vi "tprofile_testread.vi"() -> ()   [LabVIEW 2017]
uses:
  <vilib>/Utility/file.llb/Read Delimited Spreadsheet (string).vi
panel:
  out "Array 4":i32[](array[numeric])
  out "Array 3":i32[](array[numeric])
  out "Array 2":i32[](array[numeric])
  out "output array":i32[](array[numeric])
  out "Array":i32[](array[numeric])
  out "all rows":string[][](array[string])
  in  "Path":path
  in  "stop":bool
  in  "Import Profile":bool
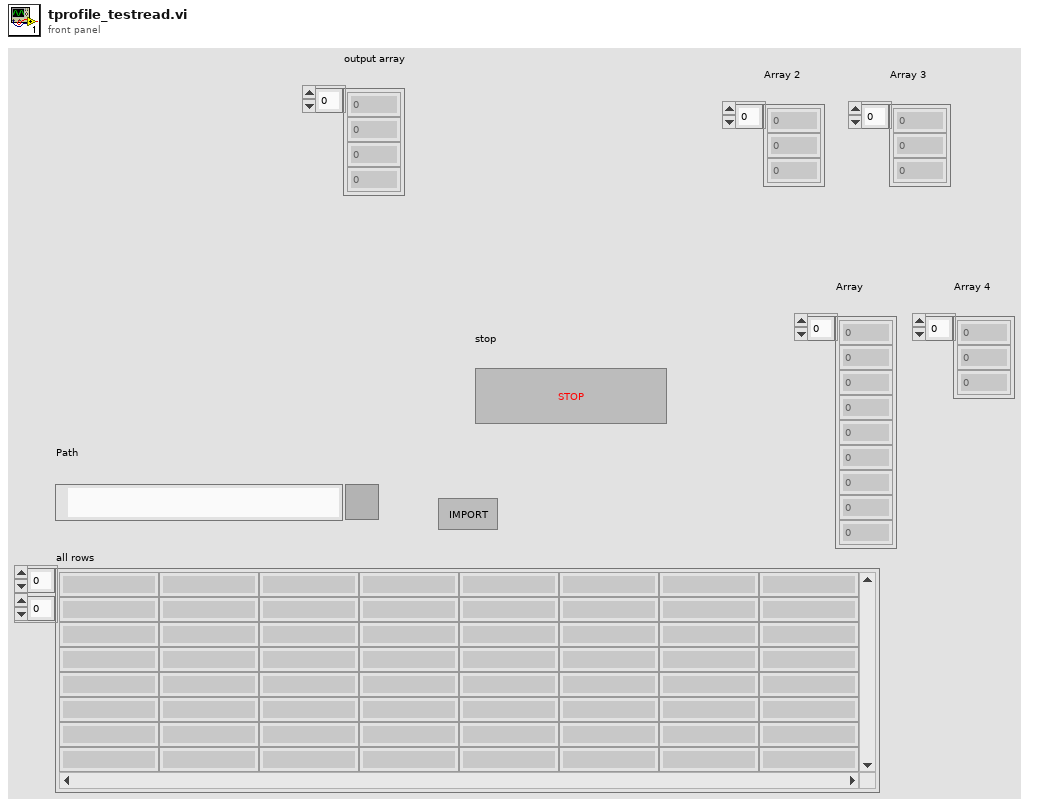
[diagram p1: front panel]
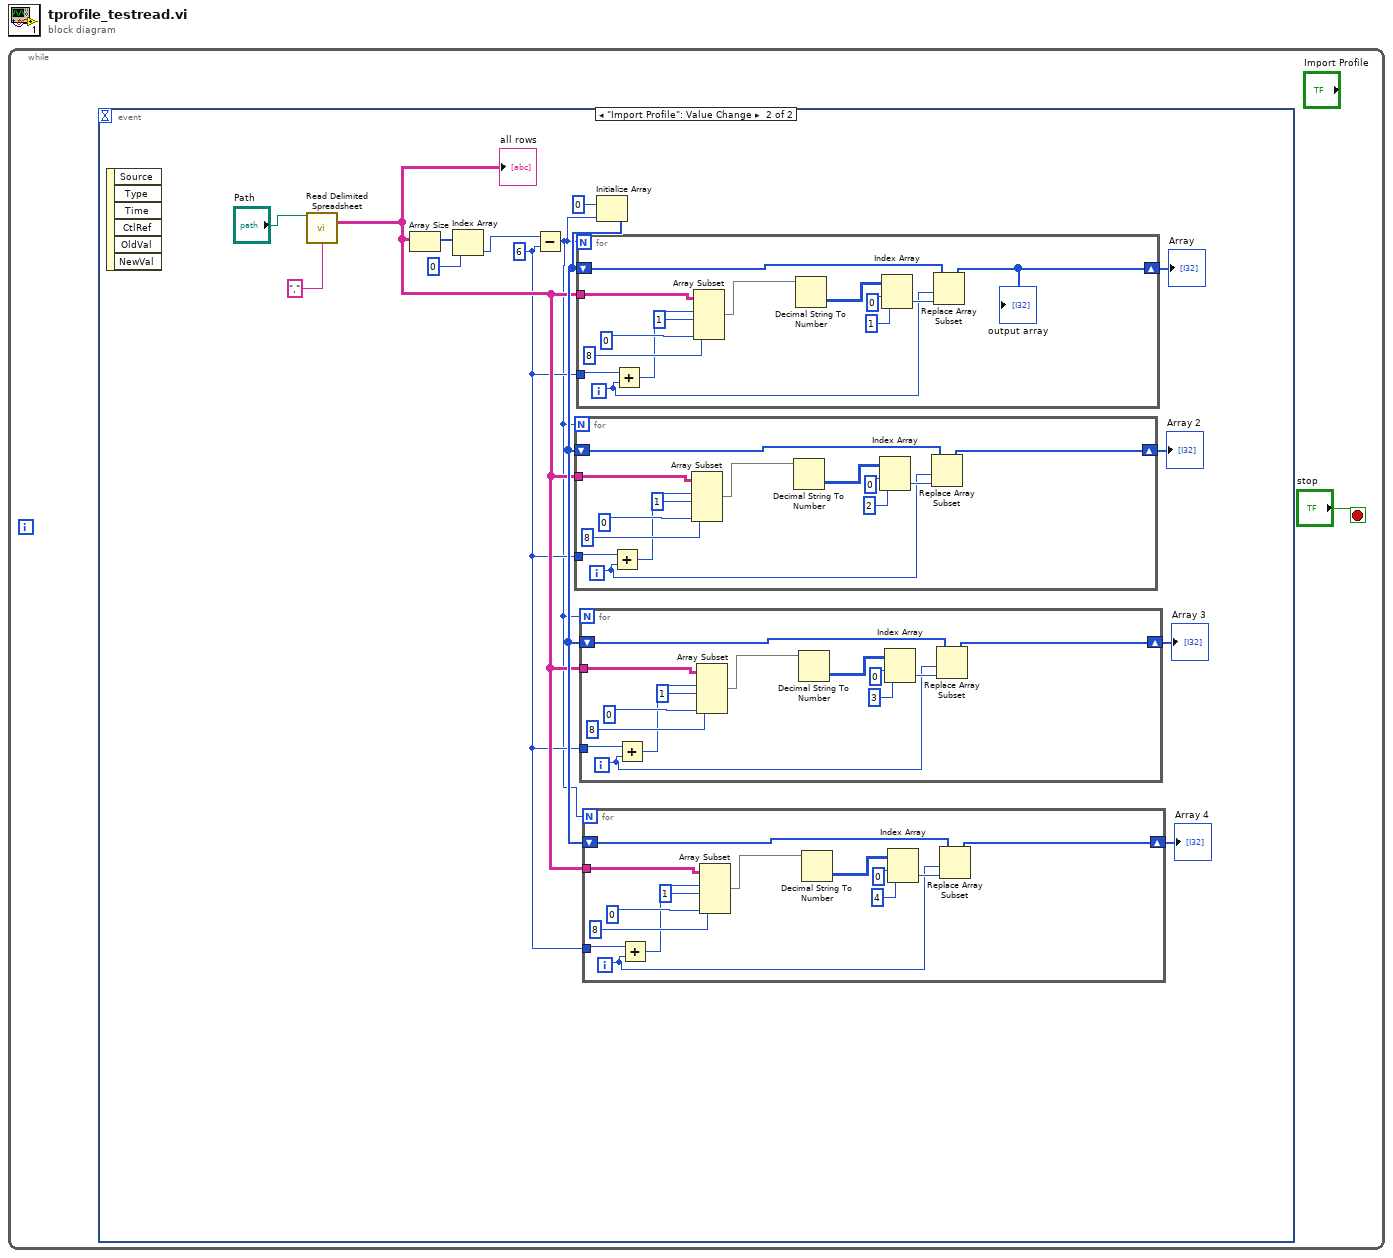
[diagram p0: block diagram]
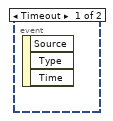
[diagram p2: hidden frame]
diagram:
  n1 = while {
    stop <- "stop" stop-if-true
    n2 = event shown="[1] \"Import Profile\": Value Change" {
      selector: _ -> [_ _]
      dyn-events: _ -> [_ _]
      timeout: _ -> [_ _]
      event Timeout {
        n3 = event-data() -> ()  [unwired: 1 in, 3 out]
      }
      event "Import Profile": Value Change {
        w3 = 6 ("Numeric")
        n4 = event-data() -> ()  [unwired: 1 in, 6 out]
        n5 = call-poly <vilib>:"Read Delimited Spreadsheet.vi"("file path (dialog if empty)"="Path", "delimiter (\\t)"="," ("delimiter (\\t)")) -> ("all rows"=w4:string[][])  [unwired: 8 in, 5 out]
        "all rows" <- w4
        n6 = Array Size(array=w4) -> (size(s)=w13:i32[])
        n7 = Index Array(array=w13, index=0) -> (element=w11:i32)
        n8 = Subtract(x=w11, y=w3) -> (x-y=w2:i32)
        n9 = Initialize Array(0, w2) -> (w5:i32[])
        n10 = for {
          N: w2 -> [_]
          tunnel: w4 -> [w57]
          tunnel: w3 -> [w52]
          shift-right: [w44] -> w8
          shift-left: w5 -> [w45]
          i -> [w47]
          n11 = Add(x=w52, y=w47) -> (x+y=w53:i32)
          n12 = Array Subset(array=w57, index (row)=w53, length (row)=1 ("length"), index (col)=0 ("index"), length (col)=8 ("length")) -> (w51:string[][])
          n13 = Decimal String To Number(string=w51) -> (number=w46:i32[][])  [unwired: 2 in, 1 out]
          n14 = Index Array(array=w46, index (row)=0, index (col)=2 ("disabled index (col)")) -> (element=w49:i32)
          n15 = Replace Array Subset(array=w45, new element=w49, index=w47) -> (w44:i32[])
        }
        "Array 2" <- w8
        n16 = for {
          N: w2 -> [_]
          tunnel: w4 -> [w71]
          tunnel: w3 -> [w66]
          shift-right: [w62] -> w9
          shift-left: w5 -> [w58]
          i -> [w60]
          n17 = Add(x=w66, y=w60) -> (x+y=w67:i32)
          n18 = Array Subset(array=w71, index (row)=w67, length (row)=1 ("length"), index (col)=0 ("index"), length (col)=8 ("length")) -> (w65:string[][])
          n19 = Decimal String To Number(string=w65) -> (number=w59:i32[][])  [unwired: 2 in, 1 out]
          n20 = Index Array(array=w59, index (row)=0, index (col)=1 ("disabled index (col)")) -> (element=w63:i32)
          n21 = Replace Array Subset(array=w58, new element=w63, index=w60) -> (w62:i32[])
          "output array" <- w62
        }
        "Array" <- w9
        n22 = for {
          N: w2 -> [_]
          tunnel: w4 -> [w43]
          tunnel: w3 -> [w38]
          shift-right: [w34] -> w7
          shift-left: w5 -> [w30]
          i -> [w32]
          n23 = Add(x=w38, y=w32) -> (x+y=w39:i32)
          n24 = Array Subset(array=w43, index (row)=w39, length (row)=1 ("length"), index (col)=0 ("index"), length (col)=8 ("length")) -> (w37:string[][])
          n25 = Decimal String To Number(string=w37) -> (number=w31:i32[][])  [unwired: 2 in, 1 out]
          n26 = Index Array(array=w31, index (row)=0, index (col)=3 ("disabled index (col)")) -> (element=w35:i32)
          n27 = Replace Array Subset(array=w30, new element=w35, index=w32) -> (w34:i32[])
        }
        "Array 3" <- w7
        n28 = for {
          N: w2 -> [_]
          tunnel: w4 -> [w29]
          tunnel: w3 -> [w24]
          shift-right: [w20] -> w6
          shift-left: w5 -> [w16]
          i -> [w18]
          n29 = Add(x=w24, y=w18) -> (x+y=w25:i32)
          n30 = Array Subset(array=w29, index (row)=w25, length (row)=1 ("length"), index (col)=0 ("index"), length (col)=8 ("length")) -> (w23:string[][])
          n31 = Decimal String To Number(string=w23) -> (number=w17:i32[][])  [unwired: 2 in, 1 out]
          n32 = Index Array(array=w17, index (row)=0, index (col)=4 ("disabled index (col)")) -> (element=w21:i32)
          n33 = Replace Array Subset(array=w16, new element=w21, index=w18) -> (w20:i32[])
        }
        "Array 4" <- w6
      }
    }
  }
